vi "Arms SSI.vi"(10 "Arms SS State":T3, 11 "Robot Controls":T4) -> (3 "Arms SS Actuator Values":T1)   [LabVIEW 2014]
uses:
  Robot Commands.ctl
  Arms SS State.ctl
  Arms SS Typedef.ctl
  <vilib>/Rock Robotics/WPI/Solenoid/WPI_SolenoidValue.ctl
panel:
  # "Field Centric"
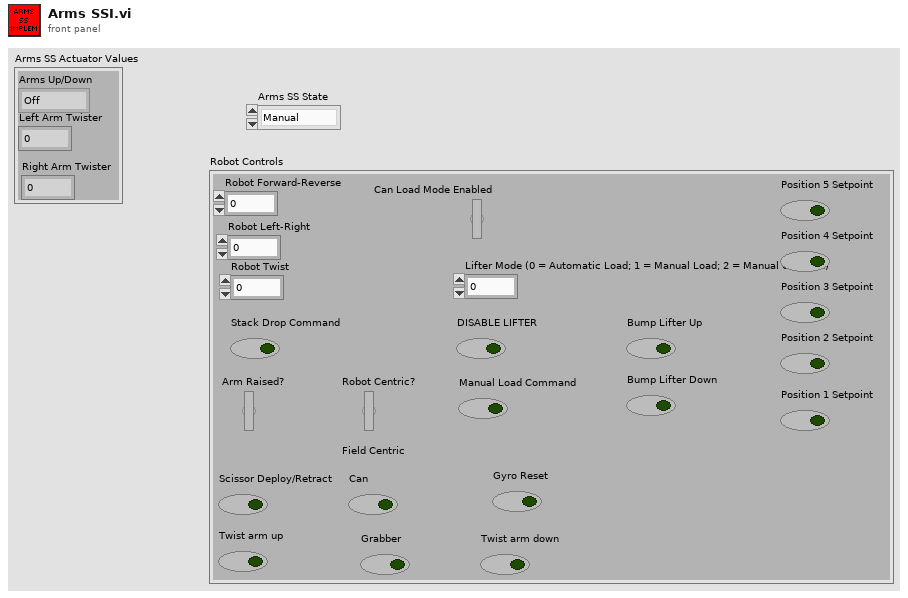
[diagram p1: front panel]
types:
  T1 = typedef "Arms SS Typedef.ctl" = cluster{"Arms Up/Down":T2, "Left Arm Twister":dbl, "Right Arm Twister":dbl}
  T2 = typedef "WPI_SolenoidValue.ctl" = enum16{"Off", "On", "Forward", "Reverse"}
  T3 = typedef "Arms SS State.ctl" = enum16{"Manual", "Retracted", "Deployed"}
  T4 = typedef "Robot Commands.ctl" = cluster{"Robot Forward-Reverse":dbl, "Robot Left-Right":dbl, "Robot Twist":dbl, "Can Load Mode Enabled":bool, "Lifter Mode (0 = Automatic Load; 1 = Manual Load; 2 = Manual Override)":dbl, "Stack Drop Command":bool, "Arm Raised?":bool, "DISABLE LIFTER":bool, "Position 1 Setpoint":bool, "Position 2 Setpoint":bool, "Position 3 Setpoint":bool, "Position 4 Setpoint":bool, "Position 5 Setpoint":bool, "Bump Lifter Down":bool, "Bump Lifter Up":bool, "Manual Load Command":bool, "Robot Centric?":bool, "Scissor Deploy/Retract":bool, "Grabber":bool, "Can":bool, "Twist arm up":bool, "Gyro Reset":bool, "Twist arm down":bool}
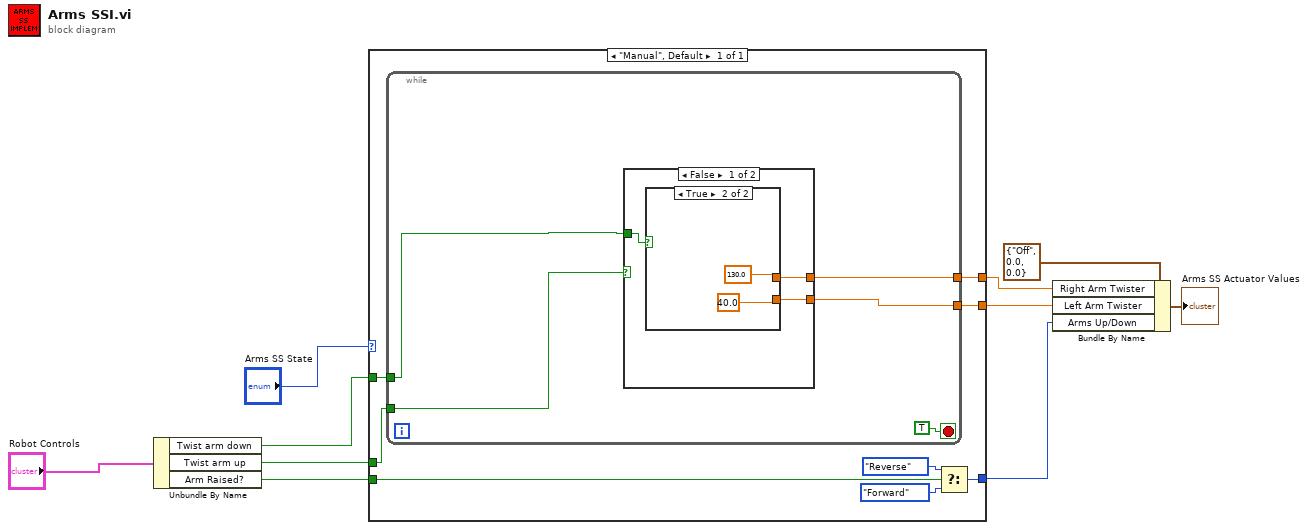
[diagram p0: block diagram]
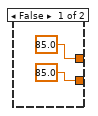
[diagram p2: hidden frame]
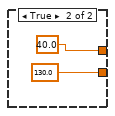
[diagram p3: hidden frame]
diagram:
  n1 = Unbundle By Name("Robot Controls") -> ("Twist arm down"=w1:bool, "Twist arm up"=w7:bool, "Arm Raised?"=w5:bool)
  n2 = case shown="\"Manual\", Default" "Arms SS State" {
    tunnel: w7 -> [w14]
    tunnel: w5 -> [w18]
    tunnel: [w17] -> w4
    tunnel: [w13] -> w3
    tunnel: [w12] -> w2
    tunnel: w1 -> [w11]
    frame "Manual", Default {
      n3 = while {
        tunnel: w14 -> [w20]
        tunnel: [w21] -> w13
        tunnel: [w22] -> w12
        tunnel: w11 -> [w19]
        stop <- TRUE stop-if-true
        n4 = case shown="False" w20 {
          tunnel: [w26 40.0] -> w22
          tunnel: [w25 130.0] -> w21
          tunnel: w19 -> [w24 _]
          frame False {
            n5 = case shown="True" w24 {
              tunnel: [85.0 130.0] -> w26
              tunnel: [85.0 40.0] -> w25
              frame False {
              }
              frame True {
              }
            }
          }
          frame True {
          }
        }
      }
      n6 = Select(t=WPI_SolenoidValue."Reverse" ("Arms Up/Down"), s=w18, f=WPI_SolenoidValue."Forward" ("Arms Up/Down")) -> (s? t:f=w17:T2)
    }
  }
  n7 = Bundle By Name(cluster=T1 {"Arms Up/Down"=enum."Off", "Left Arm Twister"=0.0, "Right Arm Twister"=0.0} ("Arms SS Actuator Values"), "Right Arm Twister"=w2, "Left Arm Twister"=w3, "Arms Up/Down"=w4) -> (→"Arms SS Actuator Values":T1)
